vi "Send Settings.vi"(8 "error in":errorcluster, 11 "ManualPS in":refnum<class "ManualPS.lvclass">) -> (0 "error out":errorcluster, 3 "ManualPS out":refnum<class "ManualPS.lvclass">)   [LabVIEW 2018, in "ManualPS.lvlib" / "ManualPS.lvclass"]
uses:
  ManualPS.lvclass
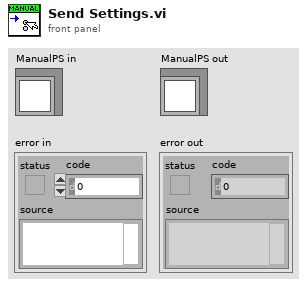
[diagram p1: front panel]
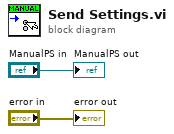
[diagram p0: block diagram]
diagram:
  "error out" <- "error in"
  "ManualPS out" <- "ManualPS in"
